vi "图像裁剪(子VI).vi"(11 "Image Pixels (U8)":u8[][](array[numeric])) -> (1 "数组":u8[][](array[numeric]), 2 "X_Left":i32, 3 "Y_Roof":i32, 4 "X_Right":i32, 5 "Y_Bottom":i32)   [LabVIEW 2012]
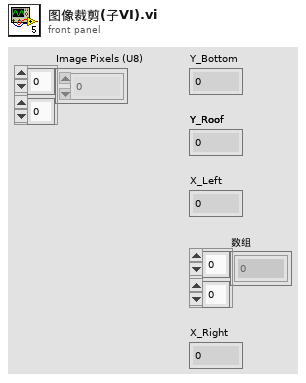
[diagram p1: front panel]
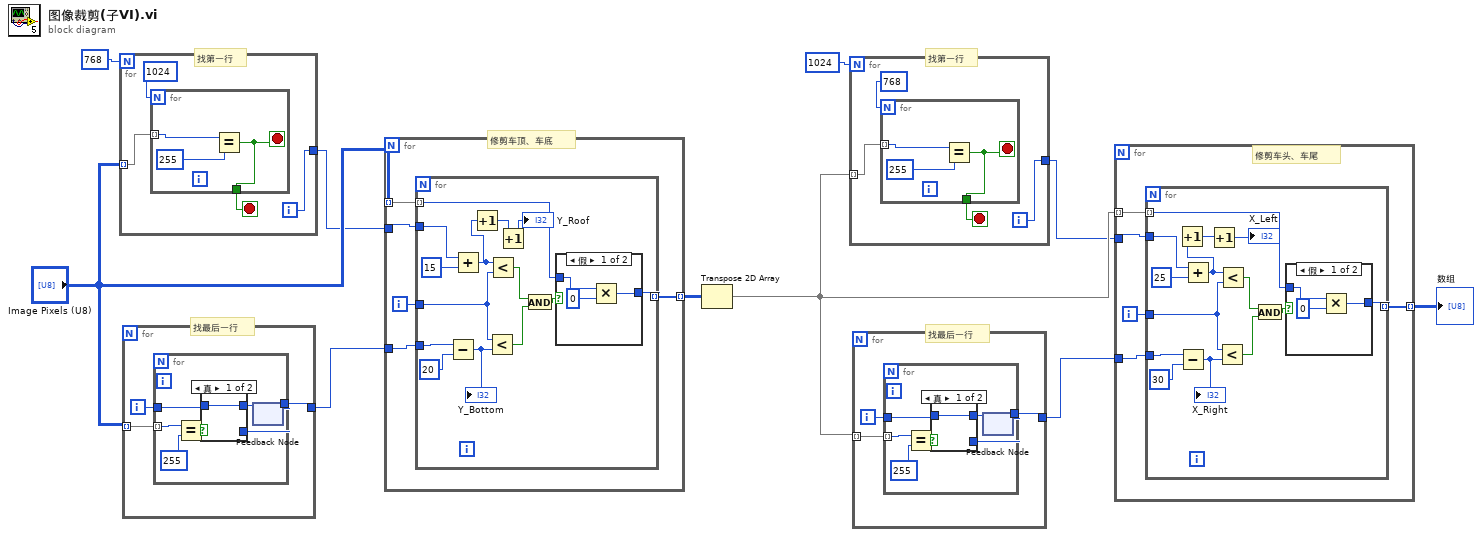
[diagram p0: block diagram]
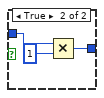
[diagram p3: hidden frame]
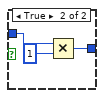
[diagram p5: hidden frame]
diagram:
  # "找最后一行"
  # "找第一行"
  # "找最后一行"
  # "找第一行"
  # "修剪车顶、车底"
  n1 = for {
    N: 768 -> [_]
    tunnel: "Image Pixels (U8)" -> [w13] mode=indexing
    tunnel: [w11] -> w2
    i -> [w11]
    stop <- w12 stop-if-true
    n2 = for {
      N: 1024 -> [_]
      tunnel: w13 -> [w16] mode=indexing
      tunnel: [w15] -> w12
      stop <- w15 stop-if-true
      n3 = Equal?(x=w16, y=u8 255) -> (x = y?=w15:bool)
    }
  }
  n4 = for {
    tunnel: "Image Pixels (U8)" -> [w20] mode=indexing
    tunnel: [w18] -> w3
    i -> [w19]
    n5 = for {
      tunnel: w20 -> [w23] mode=indexing
      tunnel: [w25] -> w18
      tunnel: w19 -> [w21]
      n6 = Equal?(x=w23, y=u8 255) -> (x = y?=w24:bool)
      n7 = feedback #1() -> (w25:i32)  [unwired: 1 in]
      n8 = case shown="真" w24 {
        tunnel: w21 -> [w27 _]
        tunnel: [w27 w28] -> w26
        tunnel: w25 -> [_ w28]
        frame True {
        }
        frame False {
        }
      }
      n9 = feedback-in #1(w26) -> ()
    }
  }
  n10 = for {
    tunnel: w2 -> [w33]
    tunnel: "Image Pixels (U8)" -> [w30] mode=indexing
    tunnel: w3 -> [w32]
    tunnel: [w29] -> w8 mode=indexing
    i -> [w31]
    n11 = for {
      tunnel: w33 -> [w39]
      tunnel: w32 -> [w46]
      tunnel: w31 -> [w42]
      tunnel: w30 -> [w37] mode=indexing
      tunnel: [w38] -> w29 mode=indexing
      n12 = Subtract(x=w46, y=20) -> (x-y=w44:i32)
      "Y_Bottom" <- w44
      n13 = Add(x=w39, y=15) -> (x+y=w36:i32)
      n14 = Increment(x=w36) -> (x+1=w35:i32)
      n15 = Less?(x=w42, y=w44) -> (x < y?=w41:bool)
      n16 = Less?(x=w36, y=w42) -> (x < y?=w43:bool)
      n17 = Increment(x=w35) -> (x+1=→"Y_Roof":i32)
      n18 = And(x=w43, y=w41) -> (x .and. y?=w40:bool)
      n19 = case shown="假" w40 {
        tunnel: w37 -> [w50 w53]
        tunnel: [w49 w51] -> w38
        frame False {
          n20 = Multiply(x=w50, y=u8 0) -> (x*y=w49:u8)
        }
        frame True {
          n21 = Multiply(x=w53, y=u8 1) -> (x*y=w51:u8)
        }
      }
    }
  }
  n22 = Transpose 2D Array(2D array=w8) -> (transposed array=w10:u8[][])
  n23 = for {
    N: 1024 -> [_]
    tunnel: w10 -> [w56] mode=indexing
    tunnel: [w54] -> w6
    i -> [w54]
    stop <- w55 stop-if-true
    n24 = for {
      N: 768 -> [_]
      tunnel: w56 -> [w59] mode=indexing
      tunnel: [w58] -> w55
      stop <- w58 stop-if-true
      n25 = Equal?(x=w59, y=u8 255) -> (x = y?=w58:bool)
    }
  }
  n26 = for {
    tunnel: w10 -> [w63] mode=indexing
    tunnel: [w61] -> w7
    i -> [w62]
    n27 = for {
      tunnel: w63 -> [w66] mode=indexing
      tunnel: [w68] -> w61
      tunnel: w62 -> [w64]
      n28 = Equal?(x=w66, y=u8 255) -> (x = y?=w67:bool)
      n29 = feedback #2() -> (w68:i32)  [unwired: 1 in]
      n30 = case shown="真" w67 {
        tunnel: w64 -> [w70 _]
        tunnel: [w70 w71] -> w69
        tunnel: w68 -> [_ w71]
        frame True {
        }
        frame False {
        }
      }
      n31 = feedback-in #2(w69) -> ()
    }
  }
  n32 = for {
    tunnel: w6 -> [w76]
    tunnel: w10 -> [w73] mode=indexing
    tunnel: w7 -> [w75]
    tunnel: [w72] -> w9 mode=indexing
    i -> [w74]
    # "修剪车头、车尾"
    n33 = for {
      tunnel: w76 -> [w82]
      tunnel: w75 -> [w89]
      tunnel: w74 -> [w85]
      tunnel: w73 -> [w80] mode=indexing
      tunnel: [w81] -> w72 mode=indexing
      n34 = Subtract(x=w89, y=30) -> (x-y=w87:i32)
      "X_Right" <- w87
      n35 = Add(x=w82, y=25) -> (x+y=w79:i32)
      n36 = Increment(x=w79) -> (x+1=w78:i32)
      n37 = Increment(x=w78) -> (x+1=→"X_Left":i32)
      n38 = Less?(x=w85, y=w87) -> (x < y?=w84:bool)
      n39 = Less?(x=w79, y=w85) -> (x < y?=w86:bool)
      n40 = And(x=w86, y=w84) -> (x .and. y?=w83:bool)
      n41 = case shown="假" w83 {
        tunnel: w80 -> [w93 w96]
        tunnel: [w92 w94] -> w81
        frame False {
          n42 = Multiply(x=w93, y=u8 0) -> (x*y=w92:u8)
        }
        frame True {
          n43 = Multiply(x=w96, y=u8 1) -> (x*y=w94:u8)
        }
      }
    }
  }
  "数组" <- w9
